vi "Adv_GetWindowsProcesses.vi"(8 "error in (no error)":errorcluster, 11 "LightField Automation in":refnum<class "LightField Automation.lvclass">) -> (0 "error out":errorcluster, 2 "AddInProcess Processes":i32[](array[numeric]), 3 "LightField Automation out":refnum<class "LightField Automation.lvclass">)   [LabVIEW 2013, in "LightField Automation.lvclass"]
uses:
  LightField Automation.lvclass
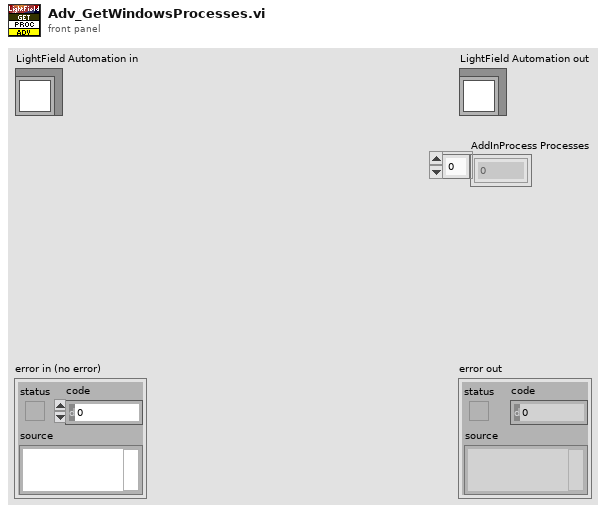
[diagram p1: front panel]
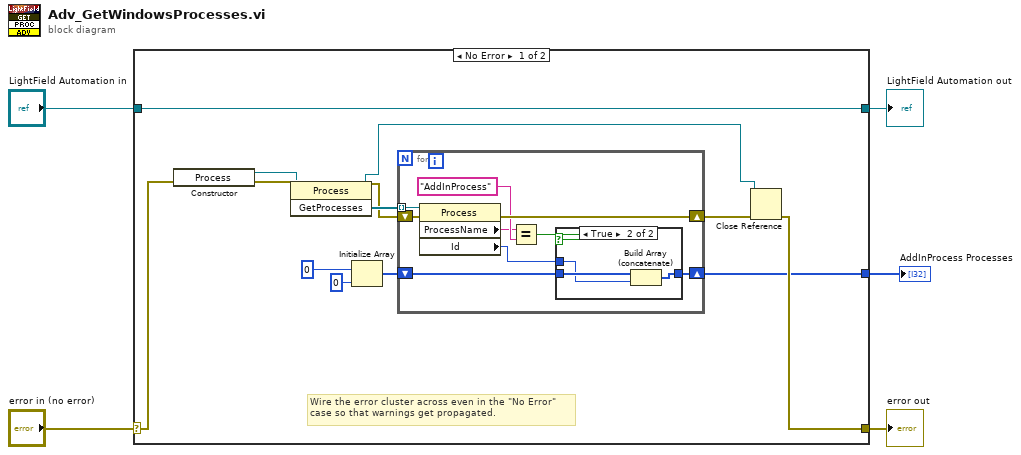
[diagram p0: block diagram]
diagram:
  n1 = case shown="No Error" "error in (no error)" {
    selector: "error in (no error)" -> [w13 w33]
    tunnel: [w12 w33] -> w4
    tunnel: [w18 w32] -> w2
    tunnel: "LightField Automation in" -> [w18 w32]
    tunnel: [w7 _] -> w1
    frame No Error {
      # "Wire the error cluster across even in the \"No Error\"\ncase so that warnings get propagated."
      n2 = constructor class="Process"(error in=w13) -> (reference out=w16:refnum<k24>, error out=w17:errorcluster)  [unwired: 2 in, 1 out]
      n3 = invoke class="Process" method="GetProcesses"(reference=w16, error in=w17) -> (reference out=w11:refnum<k24>, error out=w10:errorcluster, "GetProcesses"=w15:refnum<k24>[])  [unwired: 1 in]
      n4 = Initialize Array(0 ("Id"), 0 ("dimension size")) -> (w8:i32[])
      n5 = for {
        tunnel: w15 -> [w25] mode=indexing
        shift-right: [w26] -> w14
        shift-left: w10 -> [w27]
        shift-right: [w20] -> w7
        shift-left: w8 -> [w22]
        n6 = property class="Process"(reference=w25, error in=w27) -> (error out=w26:errorcluster, "ProcessName"=w21:string, "Id"=w19:i32)  [unwired: 1 out]
        n7 = Equal?(x=w21, y="AddInProcess") -> (x = y?=w23:bool)
        n8 = case shown="True" w23 {
          tunnel: w22 -> [w28 w31]
          tunnel: [w28 w30] -> w20
          tunnel: w19 -> [_ w29]
          frame False {
          }
          frame True {
            n9 = Build Array (concatenate)(w31, w29) -> (w30:i32[])
          }
        }
      }
      n10 = Close Reference(reference=w11, error in (no error)=w14) -> (error out=w12:errorcluster)
    }
    frame Error {
    }
  }
  "error out" <- w4
  "LightField Automation out" <- w2
  "AddInProcess Processes" <- w1
